vi "Control Voltage Level.vi"(8 "error in (no error)":errorcluster, 10 "Voltage Level (0.0 V)":dbl format="%.2g", 11 "VISA resource name":refnum<visa-resource-name>) -> (0 "error out":errorcluster, 3 "VISA resource name out":refnum<visa-resource-name>)   [LabVIEW 2020, in "MagnaDC.lvlib"]
doc: "Configures over voltage protection (OVP) of the power supply. Specify the voltage limit and whether to enable or disable OVP."
uses:
  MagnaDC.lvlib
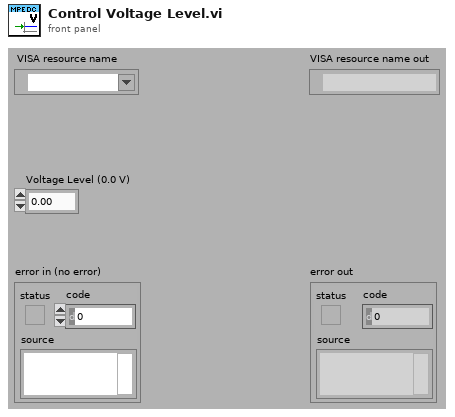
[diagram p1: front panel]
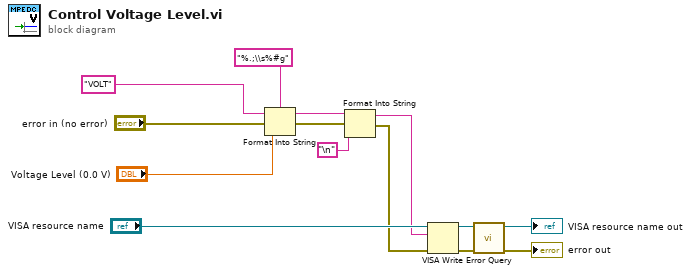
[diagram p0: block diagram]
diagram:
  n1 = Format Into String(format string="%.;\\s%#g", initial string="VOLT", error in="error in (no error)", "Voltage Level (0.0 V)") -> (resulting string=w7:string, error out=w8:errorcluster)
  n2 = Format Into String(initial string=w7, error in=w8, "\n") -> (resulting string=w2:string, error out=w1:errorcluster)  [unwired: 1 in]
  n3 = VISA Write(VISA resource name="VISA resource name", write buffer=w2, error in (no error)=w1) -> (VISA resource name out=w11:refnum<visa-resource-name>, error out=w12:errorcluster)  [unwired: 1 out]
  n4 = call "Error Query.vi"("error in (no error)"=w12, "VISA resource name"=w11) -> ("error out"=→"error out":errorcluster, "VISA resource name out"=→"VISA resource name out":refnum<visa-resource-name>)  [unwired: 6 in, 2 out]
